vi "GenerateAttackablePosition_Rook.vi"(1 "Black/White Turn (T/F)":bool, 2 "Board":i32[][](array[numeric])=[[-3, -5, -4, -1, -2, -4, -5, -3], [-6, -6, -6, -6, -6, -6, -6, -6], [0, 0, 0, 0, 0, 0, 0, 0], [0, 0, 0, 0, 0, 0, 0, 0], [0, 0, 0, 0, 0, 0, 0, 0], [0, 0, 0, 0, 0, 0, 0, 0], [6, 6, 6, 6, 6, 6, 6, 6], [3, 5, 4, 1, 2, 4, 5, 3]], 3 "pieceIndex":i32) -> (0 "AttachablePosition":bool[][](array[boolean]))   [LabVIEW 2014]
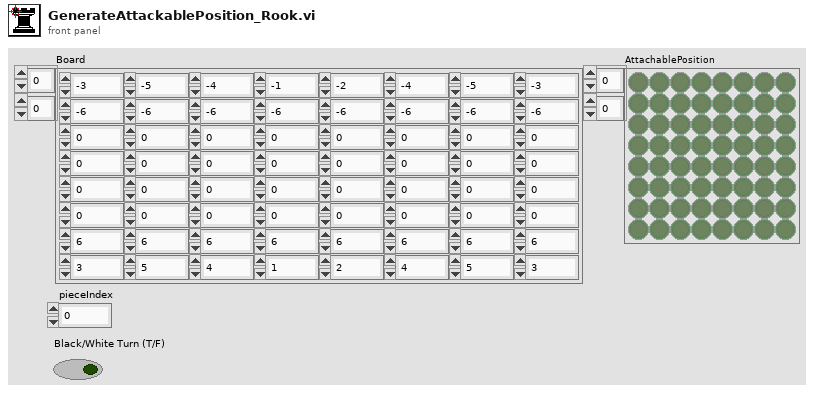
[diagram p1: front panel]
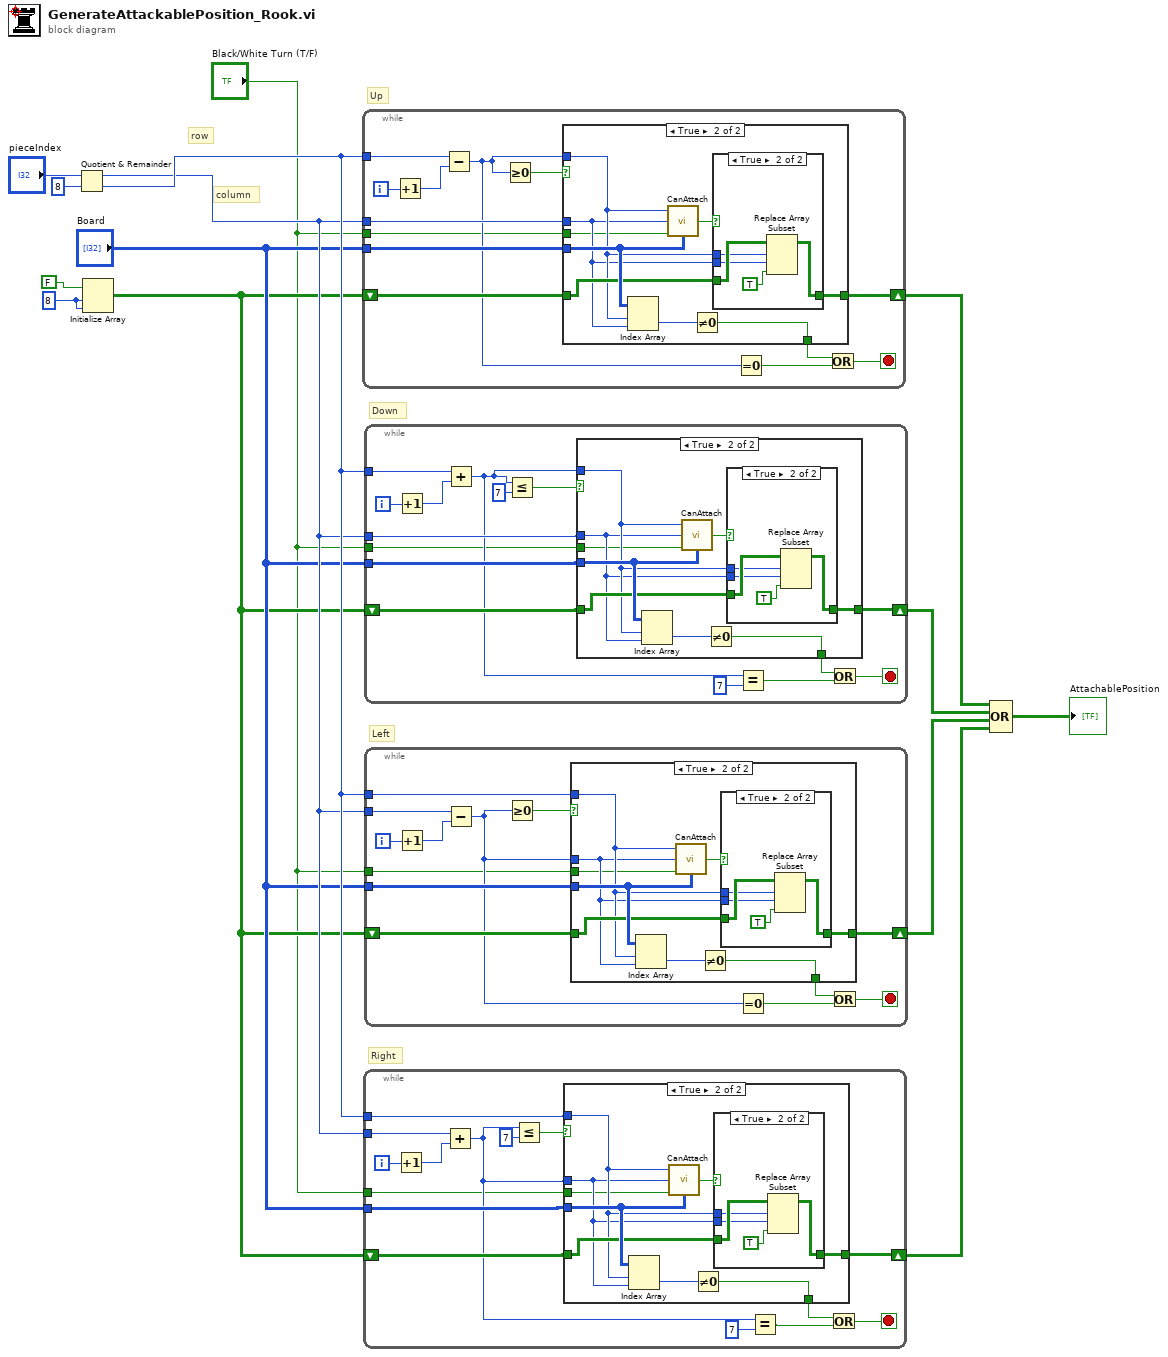
[diagram p0: block diagram]
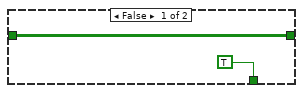
[diagram p2: hidden frame]
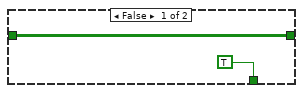
[diagram p4: hidden frame]
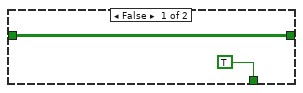
[diagram p6: hidden frame]
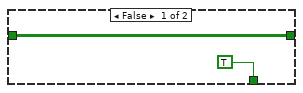
[diagram p8: hidden frame]
diagram:
  w12 = 8 ("dimension size")
  # "Right"
  # "Left"
  # "Down"
  # "Up"
  # "column"
  # "row"
  n1 = Quotient & Remainder(x="pieceIndex", y=8) -> (x-y*floor(x/y)=w4:i32, floor(x/y)=w5:i32)
  n2 = Initialize Array(FALSE, w12, w12) -> (w2:bool[][])
  n3 = while {
    tunnel: w5 -> [w25]
    tunnel: w4 -> [w19]
    tunnel: "Board" -> [w20]
    shift-right: [w22] -> w10
    shift-left: w2 -> [w21]
    tunnel: "Black/White Turn (T/F)" -> [w16]
    i -> [w27]
    stop <- w24 stop-if-true
    n4 = Increment(x=w27) -> (x+1=w26:i32)
    n5 = Subtract(x=w25, y=w26) -> (x-y=w18:i32)
    n6 = Greater Or Equal To 0?(x=w18) -> (x >= 0?=w17:bool)
    n7 = case shown="True" w17 {
      tunnel: w18 -> [_ w32]
      tunnel: w19 -> [_ w31]
      tunnel: w20 -> [_ w36]
      tunnel: w21 -> [w29 w34]
      tunnel: [w29 w33] -> w22
      tunnel: [TRUE w37] -> w15
      tunnel: w16 -> [_ w30]
      frame False {
      }
      frame True {
        n8 = Index Array(array=w36, index (row)=w32, index (col)=w31) -> (element=w38:i32)
        n9 = call "CanAttach.vi"("Board"=w36, "Black/White Turn (T/F)"=w30, "Column"=w31, "Row"=w32) -> ("Boolean"=w35:bool)
        n10 = Not Equal To 0?(x=w38) -> (x != 0?=w37:bool)
        n11 = case shown="True" w35 {
          tunnel: w34 -> [w39 w43]
          tunnel: [w39 w42] -> w33
          tunnel: w32 -> [_ w41]
          tunnel: w31 -> [_ w40]
          frame False {
          }
          frame True {
            n12 = Replace Array Subset(array=w43, new element=TRUE ("new element/subarray"), index (row)=w41, index (col)=w40) -> (w42:bool[][])
          }
        }
      }
    }
    n13 = Equal To 0?(x=w18) -> (x = 0?=w23:bool)
    n14 = Or(x=w15, y=w23) -> (x .or. y?=w24:bool)
  }
  n15 = while {
    tunnel: w5 -> [w48]
    tunnel: w4 -> [w56]
    tunnel: "Board" -> [w50]
    shift-right: [w52] -> w6
    shift-left: w2 -> [w51]
    tunnel: "Black/White Turn (T/F)" -> [w47]
    i -> [w59]
    stop <- w57 stop-if-true
    n16 = Increment(x=w59) -> (x+1=w58:i32)
    n17 = Add(x=w56, y=w58) -> (x+y=w49:i32)
    n18 = Less Or Equal?(x=w49, y=7) -> (x <= y?=w46:bool)
    n19 = case shown="True" w46 {
      tunnel: w48 -> [_ w64]
      tunnel: w49 -> [_ w63]
      tunnel: w50 -> [_ w68]
      tunnel: w51 -> [w61 w66]
      tunnel: [w61 w65] -> w52
      tunnel: [TRUE w69] -> w45
      tunnel: w47 -> [_ w62]
      frame False {
      }
      frame True {
        n20 = Index Array(array=w68, index (row)=w64, index (col)=w63) -> (element=w70:i32)
        n21 = call "CanAttach.vi"("Board"=w68, "Black/White Turn (T/F)"=w62, "Column"=w63, "Row"=w64) -> ("Boolean"=w67:bool)
        n22 = Not Equal To 0?(x=w70) -> (x != 0?=w69:bool)
        n23 = case shown="True" w67 {
          tunnel: w66 -> [w71 w75]
          tunnel: [w71 w74] -> w65
          tunnel: w64 -> [_ w73]
          tunnel: w63 -> [_ w72]
          frame False {
          }
          frame True {
            n24 = Replace Array Subset(array=w75, new element=TRUE ("new element/subarray"), index (row)=w73, index (col)=w72) -> (w74:bool[][])
          }
        }
      }
    }
    n25 = Equal?(x=w49, y=7) -> (x = y?=w54:bool)
    n26 = Or(x=w45, y=w54) -> (x .or. y?=w57:bool)
  }
  n27 = while {
    tunnel: w5 -> [w89]
    tunnel: w4 -> [w80]
    tunnel: "Board" -> [w81]
    shift-right: [w84] -> w9
    shift-left: w2 -> [w82]
    tunnel: "Black/White Turn (T/F)" -> [w78]
    i -> [w91]
    stop <- w88 stop-if-true
    n28 = Increment(x=w91) -> (x+1=w90:i32)
    n29 = Add(x=w89, y=w90) -> (x+y=w79:i32)
    n30 = Less Or Equal?(x=w79, y=7) -> (x <= y?=w77:bool)
    n31 = case shown="True" w77 {
      tunnel: w79 -> [_ w96]
      tunnel: w80 -> [_ w95]
      tunnel: w81 -> [_ w100]
      tunnel: w82 -> [w93 w98]
      tunnel: [w93 w97] -> w84
      tunnel: [TRUE w101] -> w83
      tunnel: w78 -> [_ w94]
      frame False {
      }
      frame True {
        n32 = Index Array(array=w100, index (row)=w96, index (col)=w95) -> (element=w102:i32)
        n33 = call "CanAttach.vi"("Board"=w100, "Black/White Turn (T/F)"=w94, "Column"=w95, "Row"=w96) -> ("Boolean"=w99:bool)
        n34 = Not Equal To 0?(x=w102) -> (x != 0?=w101:bool)
        n35 = case shown="True" w99 {
          tunnel: w98 -> [w103 w107]
          tunnel: [w103 w106] -> w97
          tunnel: w96 -> [_ w105]
          tunnel: w95 -> [_ w104]
          frame False {
          }
          frame True {
            n36 = Replace Array Subset(array=w107, new element=TRUE ("new element/subarray"), index (row)=w105, index (col)=w104) -> (w106:bool[][])
          }
        }
      }
    }
    n37 = Equal?(x=w79, y=7) -> (x = y?=w87:bool)
    n38 = Or(x=w83, y=w87) -> (x .or. y?=w88:bool)
  }
  n39 = while {
    tunnel: w5 -> [w111]
    tunnel: w4 -> [w117]
    tunnel: "Board" -> [w113]
    shift-right: [w116] -> w7
    shift-left: w2 -> [w114]
    tunnel: "Black/White Turn (T/F)" -> [w110]
    i -> [w121]
    stop <- w119 stop-if-true
    n40 = Increment(x=w121) -> (x+1=w120:i32)
    n41 = Subtract(x=w117, y=w120) -> (x-y=w112:i32)
    n42 = Greater Or Equal To 0?(x=w112) -> (x >= 0?=w109:bool)
    n43 = case shown="True" w109 {
      tunnel: w111 -> [_ w126]
      tunnel: w112 -> [_ w125]
      tunnel: w113 -> [_ w130]
      tunnel: w114 -> [w123 w128]
      tunnel: [w123 w127] -> w116
      tunnel: [TRUE w131] -> w115
      tunnel: w110 -> [_ w124]
      frame False {
      }
      frame True {
        n44 = Index Array(array=w130, index (row)=w126, index (col)=w125) -> (element=w132:i32)
        n45 = call "CanAttach.vi"("Board"=w130, "Black/White Turn (T/F)"=w124, "Column"=w125, "Row"=w126) -> ("Boolean"=w129:bool)
        n46 = Not Equal To 0?(x=w132) -> (x != 0?=w131:bool)
        n47 = case shown="True" w129 {
          tunnel: w128 -> [w133 w137]
          tunnel: [w133 w136] -> w127
          tunnel: w126 -> [_ w135]
          tunnel: w125 -> [_ w134]
          frame False {
          }
          frame True {
            n48 = Replace Array Subset(array=w137, new element=TRUE ("new element/subarray"), index (row)=w135, index (col)=w134) -> (w136:bool[][])
          }
        }
      }
    }
    n49 = Equal To 0?(x=w112) -> (x = 0?=w118:bool)
    n50 = Or(x=w115, y=w118) -> (x .or. y?=w119:bool)
  }
  n51 = Compound Arithmetic op=OR(w10, w9, w7, w6) -> (→"AttachablePosition":bool[][])
